vi "PH_ForceSensor.get data to modify.vi"(0 "i ref in":refnum<vi>, 3 "ms timeout (10000)":i32=10000, 5 "error in (no error)":errorcluster) -> (14 "i ref out":refnum<vi>, 16 "i attribute":T1, 17 "timed out":bool, 19 "error out":errorcluster)   [LabVIEW 2014, in "PH_ForceSensor.lvlib"]
doc: "Reads the attribute data of the object after the access to the data has been locked by the \"acquire\" method. If the attribute data has been locked already, this methods waits until the attribute data is unlocked or there is a timeout.\n\nThe attribute data must be unlocked using the methods \"release\" or \"set modified data\".\n\nLicense Agreement for this software:\n\nCopyright (C)\nGesellschaft für Schwerionenforschung, GSI\nPlanckstr. 1\n64291 Darmstadt\nGermany\n\nContact: D.Beck@gsi.de \n\nThis program is free software; you can redistribute it and/or modify it under the terms of the GNU General Public License as published by the Free Software Foundation; either version 2 of the license, or (at your option) any later version.\n\nThis program is distributed in the hope that it will be useful, but WITHOUT ANY WARRANTY; without even the implied warranty of MERCHANTABILITY or FITNESS FOR A PARTICULAR PURPOSE. See the GNU General License for more details (http://www.gnu.org).\n\nGesellschaft für Schwerionenforschung, GSI\nPlanckstr. 1, 64291 Darmstadt, Germany\nFor all questions and ideas contact: M.Richter@gsi.de, H.Brand@gsi.de or D.Beck@gsi.de.\nLast update: 17-JUN-2004"
uses:
  PH_ForceSensor.lvlib
  PH_ForceSensor.i attribute.ctl
  PH_ForceSensor.GUI Refs.ctl
  PH_ForceSensor.Dataset.ctl
  PH_ForceSensor.Ranges.ctl
  CS_Core/CSObj/CSObj.lvlib
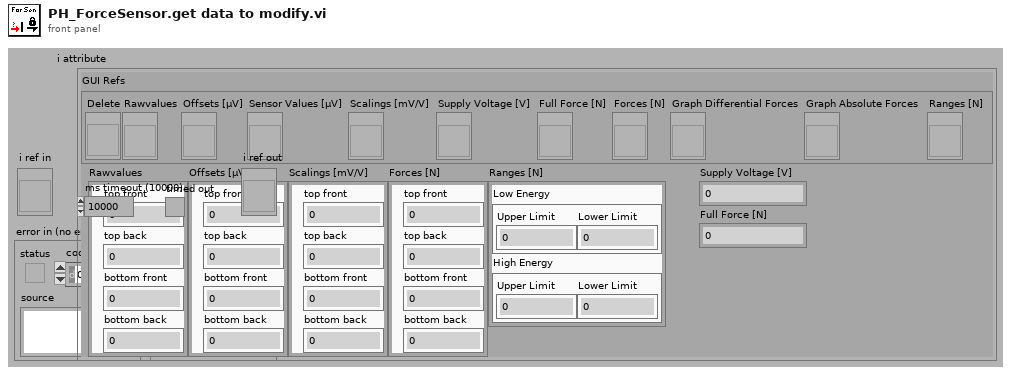
[diagram p1: front panel]
types:
  T1 = typedef "PH_ForceSensor.lvlib/PH_ForceSensor.i attribute.ctl" = cluster{"GUI Refs":T2, "Rawvalues":T3, "Offsets [µV]":T3, "Scalings [mV/V]":T3, "Forces [N]":T3, "Supply Voltage [V]":dbl, "Full Force [N]":dbl, "Ranges [N]":cluster{"Low Energy":cluster{"Upper Limit":dbl, "Lower Limit":dbl}, "High Energy":cluster{"Upper Limit":dbl, "Lower Limit":dbl}}}
  T2 = typedef "PH_ForceSensor.lvlib/PH_ForceSensor.GUI Refs.ctl" = cluster{"Delete":refnum<vi>, "Rawvalues":refnum<vi>, "Offsets [µV]":refnum<vi>, "Sensor Values [µV]":refnum<vi>, "Scalings [mV/V]":refnum<vi>, "Supply Voltage [V]":refnum<vi>, "Full Force [N]":refnum<vi>, "Forces [N]":refnum<vi>, "Graph Differential Forces":refnum<vi>, "Graph Absolute Forces":refnum<vi>, "Ranges [N]":refnum<vi>}
  T3 = typedef "PH_ForceSensor.lvlib/PH_ForceSensor.Dataset.ctl" = cluster{"top front":dbl, "top back":dbl, "bottom front":dbl, "bottom back":dbl}
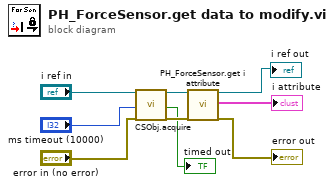
[diagram p0: block diagram]
diagram:
  n1 = call "CSObj.acquire.vi"("i ref in"="i ref in", "ms timeout (10000)"="ms timeout (10000)", "error in (no error)"="error in (no error)") -> ("i ref out"=w8:refnum<vi>, "timed out"=→"timed out":bool, "error out"=w5:errorcluster)  [unwired: 14 in]
  n2 = call "PH_ForceSensor.get i attribute.vi"("i ref in"=w8, "error in (no error)"=w5) -> ("i ref out"=→"i ref out":refnum<vi>, "i attribute"=→"i attribute":T1, "error out"=→"error out":errorcluster)  [unwired: 15 in]
